vi "Config protocol settings from meas config.vi"(11 "measurement configuration":T1={"Band start"=20.0, "Band stop"=20000.0, "Weighting Filter"=enum."Linear", "Full scale range"=2.825, "Left channel name"="", "Right channel name"="", "Left channel analog source resource name"="", "Right channel analog source resource name"="", "Frequency"=1000.0, "Amplitude"=-1.0, "Protocol capture resource name"="", "Data line"=0, "Left acquisition channel"=0, "Right acquisition channel"=0, "Sample rate"=44100.0, "Measurement Duration"=0.1, "Frame sync edge for Channel 0"=enum."Falling", "Channel count per frame"=2, "Channel length"=32, "Bit depth"=24, "Channel 0 offset"=1, "Endianness"=enum."MSB First", "Data Justification"=enum."Left Justified", "Frame length"=64, "Frame sync pulse width"=32, "Bit clock edge  sync"=enum."Falling"} {"Frame length" format="%#_6ps"}) -> (3 "Protocol settings":T2={"Protocol capture resource name"="", "Data line"=0, "Channel"="", "Clock rate"=12288000, "Number of words"=19200, "Sensitivity"=0.34762, "Frame sync edge for channel 0"=enum."Falling", "Channel count per frame"=2, "Channel length"=32, "Bit depth"=24, "Channel 0 offset"=1, "Endianness"=enum."MSB First", "Data justification"=enum."Left Justified", "Frame length"=64, "Frame sync pulse width"=32, "Bit clock edge sync"=enum."Falling"})   [LabVIEW 2021, in "AC Dual Channel_Audio ADC.lvlib"]
uses:
  AC Dual Channel_Audio ADC.lvlib
  shared/controls/Protocol Settings Dual Channel.ctl
  Measurement Configuration.ctl
  shared/controls/Audio ADC Controls.lvlib
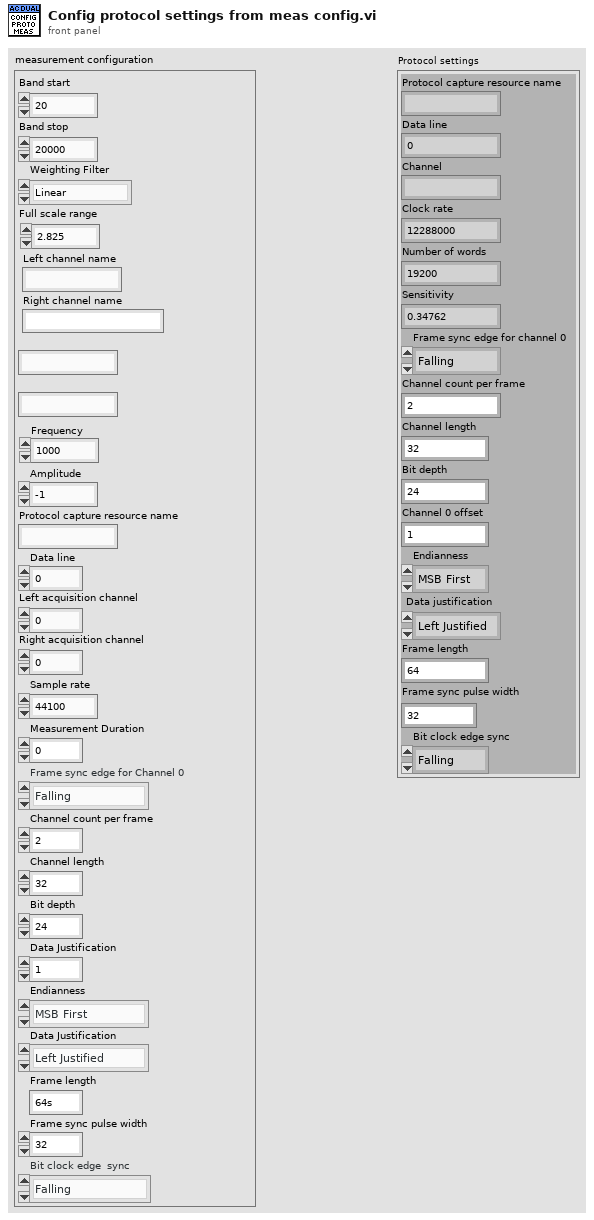
[diagram p1: front panel]
types:
  T1 = typedef "AC Dual Channel_Audio ADC.lvlib/Measurement Configuration.ctl" = cluster{"Band start":dbl, "Band stop":dbl, "Weighting Filter":enum32{"Linear", "A-weighting", "B-weighting", "C-weighting"}, "Full scale range":dbl, "Left channel name":string, "Right channel name":string, "Left channel analog source resource name":string, "Right channel analog source resource name":string, "Frequency":dbl, "Amplitude":dbl, "Protocol capture resource name":string, "Data line":i32, "Left acquisition channel":i32, "Right acquisition channel":i32, "Sample rate":dbl, "Measurement Duration":dbl, "Frame sync edge for Channel 0":enum32{"Rising", "Falling"}, "Channel count per frame":u32, "Channel length":u32, "Bit depth":u32, "Channel 0 offset":u32, "Endianness":enum32{"MSB First", "LSB First"}, "Data Justification":enum32{"Left Justified", "Right Justified"}, "Frame length":u32, "Frame sync pulse width":u32, "Bit clock edge  sync":enum32{"Rising", "Falling"}}
  T2 = typedef "Audio ADC Controls.lvlib/Protocol Settings Dual Channel.ctl" = cluster{"Protocol capture resource name":string, "Data line":u16, "Channel":string, "Clock rate":u32, "Number of words":i32, "Sensitivity":dbl, "Frame sync edge for channel 0":enum32{"Rising", "Falling"}, "Channel count per frame":u8, "Channel length":u16, "Bit depth":u8, "Channel 0 offset":u16, "Endianness":enum32{"MSB First", "LSB First"}, "Data justification":enum32{"Left Justified", "Right Justified"}, "Frame length":u16, "Frame sync pulse width":u16, "Bit clock edge sync":enum32{"Rising", "Falling"}}
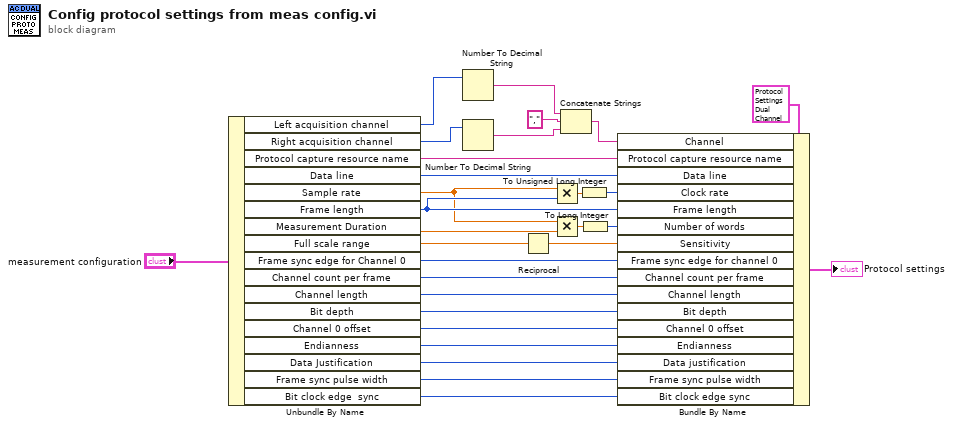
[diagram p0: block diagram]
diagram:
  n1 = Unbundle By Name("measurement configuration") -> ("Left acquisition channel"=w1:i32, "Right acquisition channel"=w7:i32, "Protocol capture resource name"=w28:string, "Data line"=w27:i32, "Sample rate"=w13:dbl, "Frame length"=w15:u32, "Measurement Duration"=w14:dbl, "Full scale range"=w10:dbl, "Frame sync edge for Channel 0"=w18:enum32{"Rising", "Falling"}, "Channel count per frame"=w26:u32, "Channel length"=w25:u32, "Bit depth"=w24:u32, "Channel 0 offset"=w23:u32, "Endianness"=w22:enum32{"MSB First", "LSB First"}, "Data Justification"=w21:enum32{"Left Justified", "Right Justified"}, "Frame sync pulse width"=w20:u32, "Bit clock edge  sync"=w19:enum32{"Rising", "Falling"})
  n2 = Number To Decimal String(number=w1) -> (decimal integer string=w5:string)  [unwired: 1 in]
  n3 = Number To Decimal String(number=w7) -> (decimal integer string=w3:string)  [unwired: 1 in]
  n4 = Reciprocal(x=w10) -> (1/x=w9:dbl)
  n5 = Multiply(x=w13, y=w15) -> (x*y=w17:dbl)
  n6 = Multiply(x=w13, y=w14) -> (x*y=w12:dbl)
  n7 = Concatenate Strings(w5, "," ("string"), w3) -> (w6:string)
  n8 = To Unsigned Long Integer(number=w17) -> (unsigned 32bit integer=w16:u32)
  n9 = To Long Integer(number=w12) -> (32bit integer=w11:i32)
  n10 = Bundle By Name(cluster=T2 {"Protocol capture resource name"="", "Data line"=0, "Channel"="", "Clock rate"=12288000, "Number of words"=19200, "Sensitivity"=0.34762, "Frame sync edge for channel 0"=enum."Falling", "Channel count per frame"=2, "Channel length"=32, "Bit depth"=24, "Channel 0 offset"=1, "Endianness"=enum."MSB First", "Data justification"=enum."Left Justified", "Frame length"=64, "Frame sync pulse width"=32, "Bit clock edge sync"=enum."Falling"} ("Protocol settings"), "Channel"=w6, "Protocol capture resource name"=w28, "Data line"=w27, "Clock rate"=w16, "Frame length"=w15, "Number of words"=w11, "Sensitivity"=w9, "Frame sync edge for channel 0"=w18, "Channel count per frame"=w26, "Channel length"=w25, "Bit depth"=w24, "Channel 0 offset"=w23, "Endianness"=w22, "Data justification"=w21, "Frame sync pulse width"=w20, "Bit clock edge sync"=w19) -> (→"Protocol settings":T2)
